vi "RP Read Status.vi"   [LabVIEW 2015]
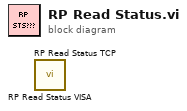
[diagram p0: block diagram]
diagram:
  n1 = call "RP Read Status VISA.vi"() -> ()  [unwired: 9 in, 3 out]
  n2 = call "RP Read Status TCP.vi"() -> ()  [unwired: 9 in, 3 out]
